vi "Hardware Device Get All Info.vi"(8 "error in":errorcluster, 9 "Terminals":tag[](array[tag]), 11 "NI PWM Input in":refnum<class "NI PWM Input.lvclass">) -> (0 "error out":errorcluster, 1 "CI.PhysicalChans":tag[](array[tag]), 3 "NI PWM Input out":refnum<class "NI PWM Input.lvclass">)   [LabVIEW 2023, in "HardwareAbstractionLayer_LVOOP.lvlib" / "NI PWM Input.lvclass"]
doc: "This VI is AI Physical Channel Read"
uses:
  NI PWM Input.lvclass
  NI PWM Input.lvclass/NI PWM Input.ctl
  <resource>/objmgr/daqmx.rc
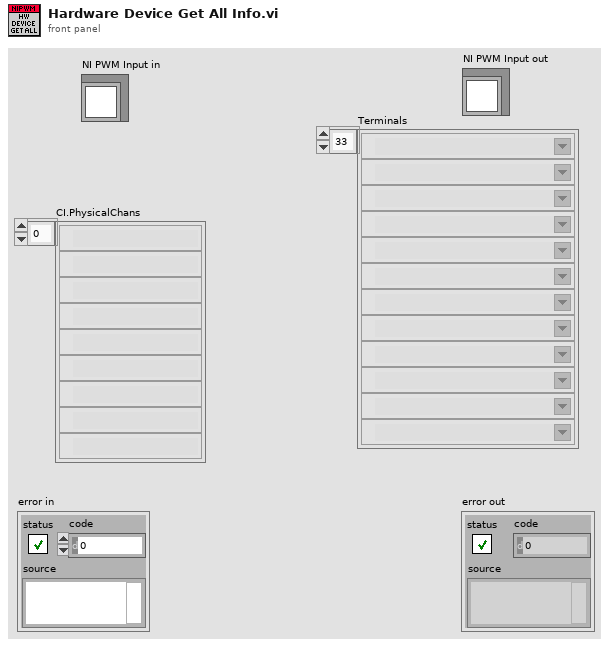
[diagram p1: front panel]
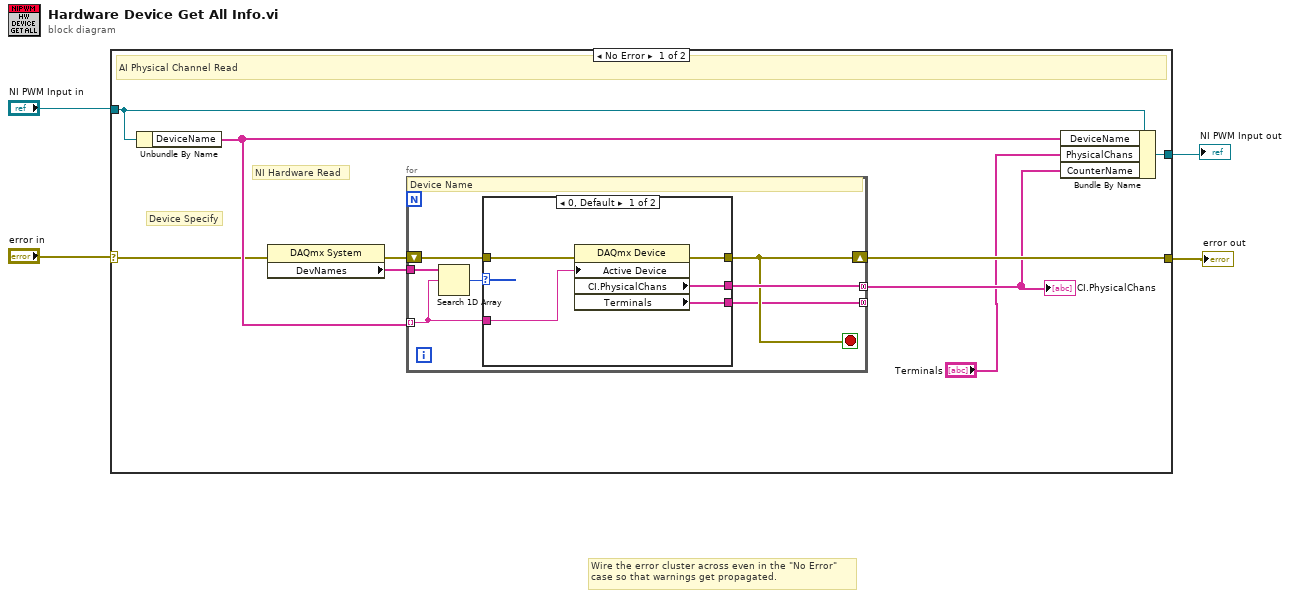
[diagram p0: block diagram]
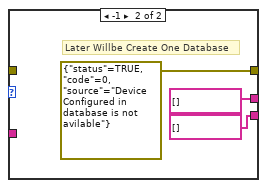
[diagram p2: hidden frame]
diagram:
  # "Wire the error cluster across even in the \"No Error\"\ncase so that warnings get propagated."
  n1 = case shown="No Error" "error in" {
    selector: "error in" -> [w7 w30]
    tunnel: [w8 w30] -> w3
    tunnel: [w13 w29] -> w1
    tunnel: "NI PWM Input in" -> [w12 w29]
    frame No Error {
      # "Device Specify"
      # "NI Hardware Read"
      # "AI Physical Channel Read"
      n2 = Unbundle By Name(w12) -> ("DeviceName"=w11:tag[])
      n3 = property class="DAQmx System"(error in=w7) -> (error out=w9:errorcluster, "DevNames"=w10:tag[])  [unwired: 1 in, 1 out]
      n4 = for {
        tunnel: w11 -> [w17] mode=indexing
        tunnel: w10 -> [w18]
        tunnel: [w16] -> w6 mode=concatenating
        shift-right: [w15] -> w8
        shift-left: w9 -> [w19]
        tunnel: [w14] -> _ mode=concatenating
        stop <- w15 stop-if-true
        # "Device Name"
        n5 = Search 1D Array(1D array=w18, element=w17) -> (index of element=w20:i32)  [unwired: 1 in]
        n6 = case shown="0, Default" w20 {
          tunnel: w19 -> [w24 _]
          tunnel: [w23 errorcluster {"status"=TRUE, "code"=0, "source"="Device  Configured in database is not avilable"} ("error out")] -> w15
          tunnel: w17 -> [w22 _]
          tunnel: [w25 tag[] [] ("AI.PhysicalChans")] -> w16
          tunnel: [w21 tag[] [] ("Terminals")] -> w14
          frame 0, Default {
            n7 = property class="DAQmx Device"(error in=w24, "Active Device"=w22) -> (error out=w23:errorcluster, "CI.PhysicalChans"=w25:tag[], "Terminals"=w21:tag[])  [unwired: 1 in, 1 out]
          }
          frame -1 {
            # "Later Willbe Create One Database"
          }
        }
      }
      "CI.PhysicalChans" <- w6
      n8 = Bundle By Name(cluster=w12, "DeviceName"=w11, "PhysicalChans"="Terminals", "CounterName"=w6) -> (w13:refnum<class "NI PWM Input.lvclass">)
    }
    frame Error {
    }
  }
  "error out" <- w3
  "NI PWM Input out" <- w1
